vi "Apply Connection.vi"(8 "error in (no error)":errorcluster, 9 "Output Index":i32, 10 "Input Index":i32, 11 "Mux in":refnum<class "Mux.lvclass">) -> (0 "error out":errorcluster, 3 "Mux out":refnum<class "Mux.lvclass">)   [LabVIEW 2022 SP3, in "VideoMux.lvlib" / "Mux.lvclass"]
uses:
  Mux.lvclass
  <vilib>/IlluminatedG/lv-stream/stream/Stream.lvclass/Stream.ctl
  Mux.lvclass/Mux.ctl
  <vilib>/IlluminatedG/lv-stream/stream/Dispatch Sniffer Data.vi
  <vilib>/IlluminatedG/lv-stream/stream/Prepared.vi
  <vilib>/IlluminatedG/lv-stream/Endpoint/Cast Sniffer Callback.vi
  <vilib>/Utility/error.llb/Error Cluster From Error Code.vi
  <vilib>/IlluminatedG/lv-stream/stream/Stream.lvclass
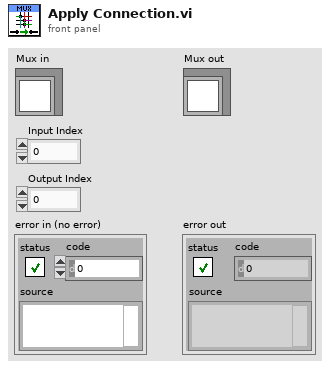
[diagram p1: front panel]
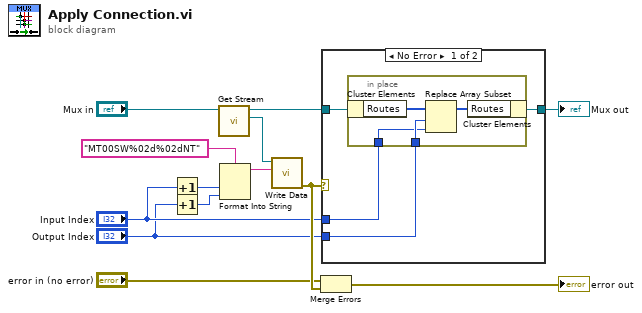
[diagram p0: block diagram]
diagram:
  n1 = Increment(x="Input Index") -> (x+1=w12:i32)
  n2 = Increment(x="Output Index") -> (x+1=w11:i32)
  n3 = call "Get Stream.vi"("Mux in"="Mux in") -> ("Stream"=w8:refnum<class "Stream.lvclass">, "Mux out"=w2:refnum<class "Mux.lvclass">)  [unwired: 8 in, 1 out]
  n4 = Format Into String(format string="MT00SW%02d%02dNT", w12, w11) -> (resulting string=w10:string)  [unwired: 2 in, 1 out]
  n5 = call <vilib>:"Write Data.vi"("Data"=w10, "Stream in"=w8) -> ("error out"=w7:errorcluster)  [unwired: 8 in, 1 out]
  n6 = Merge Errors("error in (no error)", w7) -> (→"error out":errorcluster)
  n7 = case shown="No Error" w7 {
    tunnel: "Input Index" -> [w15 _]
    tunnel: "Output Index" -> [w16 _]
    tunnel: w2 -> [w17 w22]
    tunnel: [w14 w22] -> w1
    frame No Error {
      n8 = in-place {
        in-place-border: w16 -> [w20]
        in-place-border: w15 -> [w19]
        n9 = in-place-cluster #1(w17) -> ("Routes"=w21:i32[])
        n10 = Replace Array Subset(array=w21, new element=w19, index=w20) -> (w18:i32[])
        n11 = in-place-cluster #1("Routes"=w18) -> (w14:refnum<class "Mux.lvclass">)
      }
    }
    frame Error {
    }
  }
  "Mux out" <- w1
